vi "TSC Material Boolean Type--global.vi"() -> (2 "boolean types":string[](array[string]))   [LabVIEW 2021]
doc: "Variable to hold the options for the Boolean Types for the buttons. This is used when coloring the UI to figure out how to apply the correct layers of six-color button options.\n\n<b>Code Developed By:</b>\nTechnology Service Corporation\n1983 S Liberty Drive\nBloomington, IN 47403\nwww.tsc.com/atcs\n\nDeveloper:\nDaniel Coons"
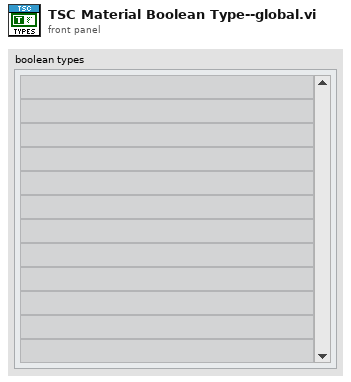
[diagram p1: front panel]
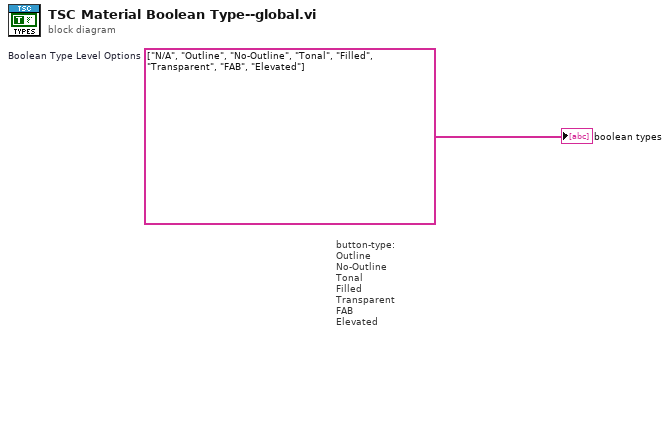
[diagram p0: block diagram]
diagram:
  w1 = string[] ["N/A", "Outline", "No-Outline", "Tonal", "Filled", "Transparent", "FAB", "Elevated"]  # Boolean Type Level Options
  # "button-type:\nOutline\nNo-Outline\nTonal\nFilled\nTransparent\nFAB\nElevated"
  "boolean types" <- w1
